vi "TestInfoCount.vi"(8 "TestResult":bool=TRUE, 11 "TestInfo out输入":T1) -> (3 "TestInfo out输出":T1)   [LabVIEW 2017]
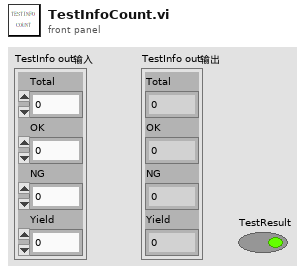
[diagram p1: front panel]
types:
  T1 = cluster{"Total":i32, "OK":i32, "NG":i32, "Yield":dbl}
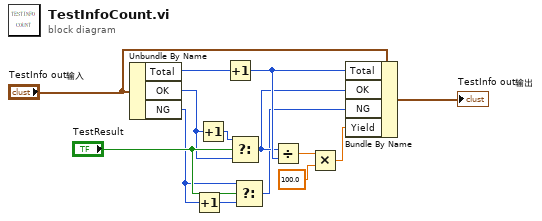
[diagram p0: block diagram]
diagram:
  n1 = Unbundle By Name("TestInfo out输入") -> ("Total"=w2:i32, "OK"=w6:i32, "NG"=w7:i32)
  n2 = Increment(x=w7) -> (x+1=w1:i32)
  n3 = Increment(x=w6) -> (x+1=w5:i32)
  n4 = Increment(x=w2) -> (x+1=w12:i32)
  n5 = Select(t=w5, s="TestResult", f=w6) -> (s? t:f=w11:i32)
  n6 = Select(t=w7, s="TestResult", f=w1) -> (s? t:f=w8:i32)
  n7 = Divide(x=w11, y=w12) -> (x/y=w10:dbl)
  n8 = Multiply(x=w10, y=100.0) -> (x*y=w9:dbl)
  n9 = Bundle By Name(cluster="TestInfo out输入", "Total"=w12, "OK"=w11, "NG"=w8, "Yield"=w9) -> (→"TestInfo out输出":T1)
